vi "Configure List Step Parameters.vi"(6 "Step Slew Rate (1)":dbl=1.0 min=0.0001 max=65536.0 step=0.0001 format="%.4g", 7 "Step Number (1)":dbl=1.0 min=1.0 max=84.0 step=1.0 format="%.0g", 8 "error in (no error)":errorcluster, 9 "Step Width (1)":dbl=1.0 min=2e-05 max=1.0 step=1e-05 format="%.5g", 10 "Step Level (1)":dbl=1.0 min=1.0 max=240.0 step=0.01 format="%.4g", 11 "VISA resource name":refnum<visa-resource-name>) -> (0 "error out":errorcluster, 3 "VISA resource name out":refnum<visa-resource-name>)   [LabVIEW 2015, in "IT8900A-E.lvlib"]
doc: "The set Vi sets the current, time width, and slope values for each step.<b>Note:</b> the current value is less than (List Range), and the slope value is changed according to (List Range). The value Range of large voltage is 0.01-3, while the value Range of small voltage is 0.001-0.3."
uses:
  <instrlib>/IT8900/IT8900A-E.lvlib
panel:
  # "s"
  # "A"
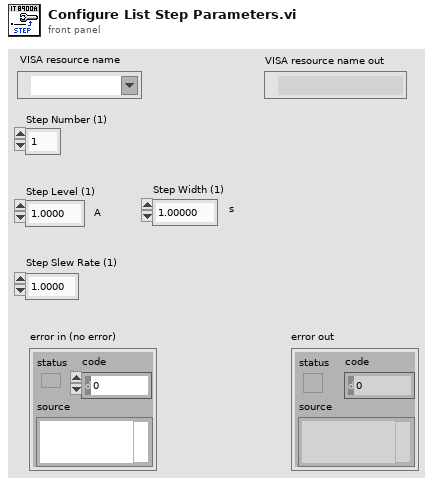
[diagram p1: front panel]
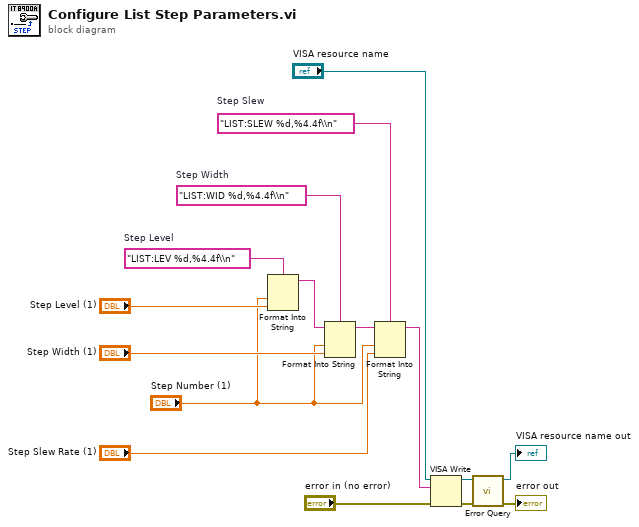
[diagram p0: block diagram]
diagram:
  w16 = "LIST:LEV %d,%4.4f\\n"  # Step Level
  w14 = "LIST:SLEW %d,%4.4f\\n"  # Step Slew
  w15 = "LIST:WID %d,%4.4f\\n"  # Step Width
  n1 = Format Into String(format string=w16, "Step Number (1)", "Step Level (1)") -> (resulting string=w9:string)  [unwired: 2 in, 1 out]
  n2 = Format Into String(format string=w15, initial string=w9, "Step Number (1)", "Step Width (1)") -> (resulting string=w8:string)  [unwired: 1 in, 1 out]
  n3 = Format Into String(format string=w14, initial string=w8, "Step Number (1)", "Step Slew Rate (1)") -> (resulting string=w1:string)  [unwired: 1 in, 1 out]
  n4 = VISA Write(VISA resource name="VISA resource name", write buffer=w1, error in (no error)="error in (no error)") -> (VISA resource name out=w5:refnum<visa-resource-name>, error out=w4:errorcluster)  [unwired: 1 out]
  n5 = call <instrlib>:"Error Query.vi"("error in (no error)"=w4, "VISA resource name"=w5) -> ("error out"=→"error out":errorcluster, "VISA resource name out"=→"VISA resource name out":refnum<visa-resource-name>)  [unwired: 6 in, 2 out]
